vi "Do.vi"(8 "error in (no error)":errorcluster, 10 "Actor in":refnum<class "Actor.lvclass">, 11 "Updata Msg":refnum<class "Updata Msg.lvclass">) -> (0 "error out":errorcluster, 2 "Actor out":refnum<class "Actor.lvclass">)   [LabVIEW 2013, in "Updata Msg.lvclass"]
doc: "This VI delivers the message to the actor by calling the appropriate method(s) on the actor."
uses:
  Updata Msg.lvclass
  <vilib>/ActorFramework/Actor/Actor.lvclass
  Display.lvclass/DisplayUI.lvclass
  Updata Msg.lvclass/Updata Msg.ctl
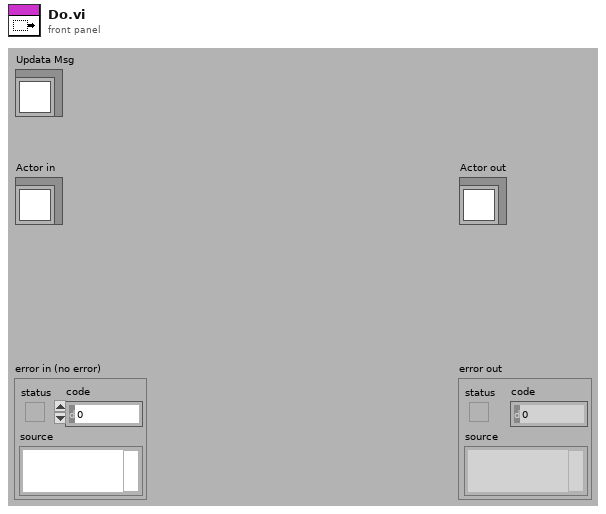
[diagram p1: front panel]
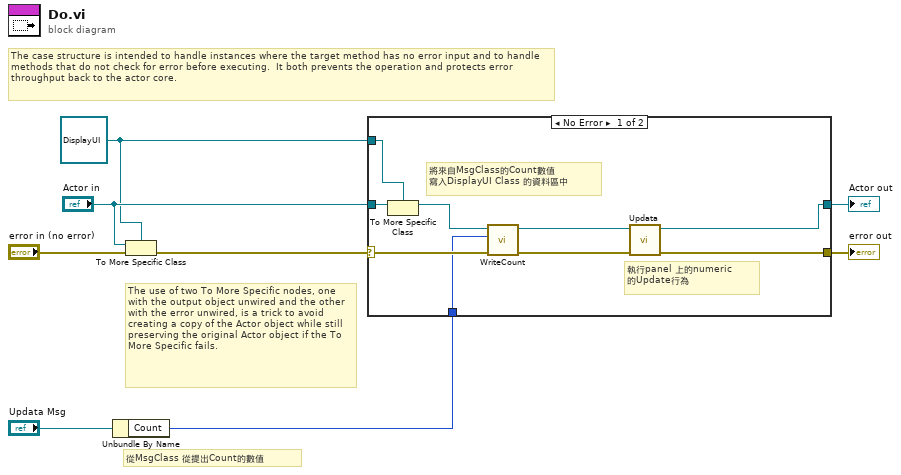
[diagram p0: block diagram]
diagram:
  w3 = refnum<class "DisplayUI.lvclass"> refnum ("Actor in")
  # "從MsgClass 從提出Count的數值"
  # "The use of two To More Specific nodes, one with the output object unwired and the other with the error unwired, is a trick to avoid creating a copy of the Actor object while still preserving the original Actor object if the To More Specific fails."
  # "The case structure is intended to handle instances where the target method has no error input and to handle methods that do not check for error before executing.  It both prevents the operation and protects error throughput back to the actor core."
  n1 = Unbundle By Name("Updata Msg") -> ("Count"=w1:i32)
  n2 = To More Specific Class(target class=w3, reference="Actor in", error in="error in (no error)") -> (error out=w7:errorcluster)  [unwired: 1 out]
  n3 = case shown="No Error" w7 {
    selector: w7 -> [w11 w19]
    tunnel: [w17 w19] -> w6
    tunnel: [w16 w18] -> w5
    tunnel: "Actor in" -> [w15 w18]
    tunnel: w3 -> [w14 _]
    tunnel: w1 -> [w9 _]
    frame No Error {
      # "執行panel 上的numeric \n的Update行為"
      # "將來自MsgClass的Count數值\n寫入DisplayUI Class 的資料區中"
      n4 = To More Specific Class(target class=w14, reference=w15) -> (specific class reference=w13:refnum<class "DisplayUI.lvclass">)  [unwired: 1 in, 1 out]
      n5 = call-dynamic "WriteCount.vi"("error in (no error)"=w11, "Count"=w9, "DisplayUI in"=w13) -> ("error out"=w10:errorcluster, "DisplayUI out"=w12:refnum<class "DisplayUI.lvclass">)  [unwired: 7 in]
      n6 = call-dynamic "Updata.vi"("error in (no error)"=w10, "DisplayUI in"=w12) -> ("error out"=w17:errorcluster, "DisplayUI out"=w16:refnum<class "DisplayUI.lvclass">)  [unwired: 8 in]
    }
    frame Error {
      # "If type check fails, pass the original object out again."
    }
  }
  "error out" <- w6
  "Actor out" <- w5
